vi "语言转化.vi"(1 "选择":i16) -> (0 "语言":string)   [LabVIEW 2014]
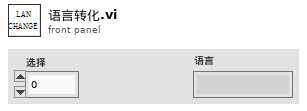
[diagram p1: front panel]
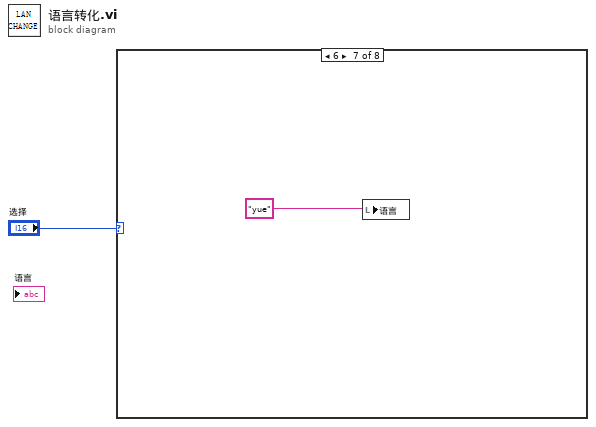
[diagram p0: block diagram]
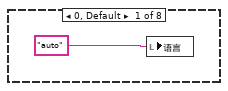
[diagram p2: hidden frame]
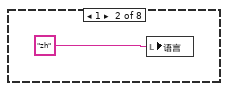
[diagram p3: hidden frame]
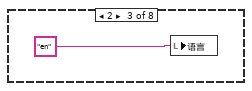
[diagram p4: hidden frame]
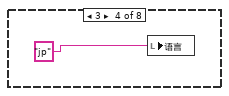
[diagram p5: hidden frame]
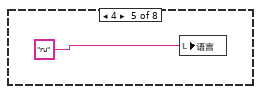
[diagram p6: hidden frame]
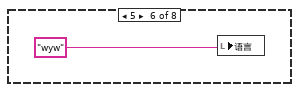
[diagram p7: hidden frame]
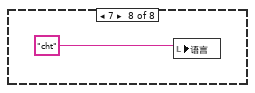
[diagram p8: hidden frame]
diagram:
  n1 = case shown="6" "选择" {
    frame 0, Default {
      n2 = local write "语言"("auto") -> ()
    }
    frame 1 {
      n3 = local write "语言"("zh") -> ()
    }
    frame 2 {
      n4 = local write "语言"("en") -> ()
    }
    frame 3 {
      n5 = local write "语言"("jp") -> ()
    }
    frame 4 {
      n6 = local write "语言"("ru") -> ()
    }
    frame 5 {
      n7 = local write "语言"("wyw") -> ()
    }
    frame 6 {
      n8 = local write "语言"("yue") -> ()
    }
    frame 7 {
      n9 = local write "语言"("cht") -> ()
    }
  }
